vi "Teleop Climb Control.vi"(9 "D-Pad":T1, 10 "Axes":T2, 11 "Button Cluster":T3) -> ()   [LabVIEW 2015]
uses:
  Common Code/Gamepads/Button Cluster.ctl
  Common Code/Gamepads/Axes Cluster.ctl
  Common Code/Gamepads/D-Pad.ctl
  Common Code/Climb Control.ctl
  Common Code/Change Detect.vi
  Common Code/Change Detect Boolean.vi
  Robot Global Data.vi
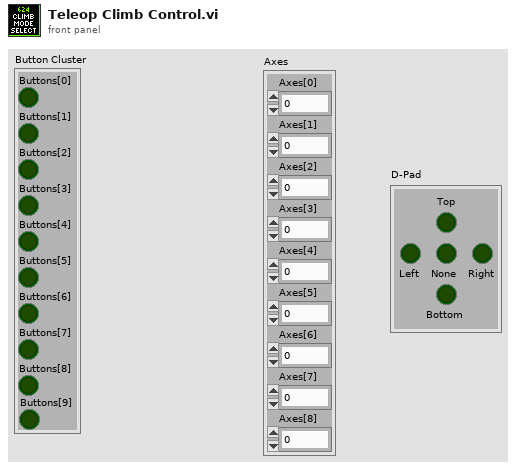
[diagram p1: front panel]
types:
  T1 = typedef "D-Pad.ctl" = cluster{"Top":bool, "Bottom":bool, "None":bool, "Right":bool, "Left":bool}
  T2 = typedef "Axes Cluster.ctl" = cluster{"Axes[0]":dbl, "Axes[1]":dbl, "Axes[2]":dbl, "Axes[3]":dbl, "Axes[4]":dbl, "Axes[5]":dbl, "Axes[6]":dbl, "Axes[7]":dbl, "Axes[8]":dbl}
  T3 = typedef "Button Cluster.ctl" = cluster{"Buttons[0]":bool, "Buttons[1]":bool, "Buttons[2]":bool, "Buttons[3]":bool, "Buttons[4]":bool, "Buttons[5]":bool, "Buttons[6]":bool, "Buttons[7]":bool, "Buttons[8]":bool, "Buttons[9]":bool}
  T4 = typedef "Climb Control.ctl" = cluster{"Climb?":bool, "Auto?":bool, "Extend":bool, "Fire":bool, "Winch\nRate":dbl}
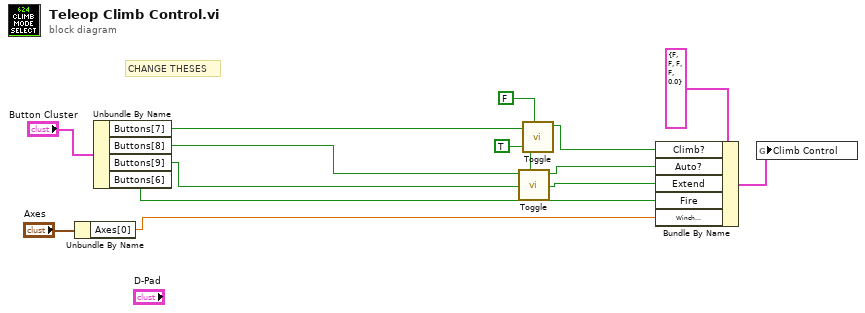
[diagram p0: block diagram]
diagram:
  # "CHANGE THESES"
  n1 = Unbundle By Name("Axes") -> ("Axes[0]"=w3:dbl)
  n2 = Unbundle By Name("Button Cluster") -> ("Buttons[7]"=w12:bool, "Buttons[8]"=w4:bool, "Buttons[9]"=w2:bool, "Buttons[6]"=w1:bool)
  n3 = call "Toggle.vi"("Initial Value"=TRUE, "In"=w4) -> ("Toggled"=w5:bool)  [unwired: 9 in]
  n4 = call "Toggle.vi"("Initial Value"=FALSE, "In"=w12) -> ("Toggled"=w7:bool)  [unwired: 9 in]
  n5 = Bundle By Name(cluster=T4 {"Climb?"=FALSE, "Auto?"=FALSE, "Extend"=FALSE, "Fire"=FALSE, "Winch\nRate"=0.0} ("Climb Control"), "Climb?"=w7, "Auto?"=w5, "Extend"=w2, "Fire"=w1, "Winch\nRate"=w3) -> (w9:T4)
  n6 = global write "Robot Global Data.vi" "Climb Control"(w9) -> ()
